vi "_API_BINANCE_GET_USDT_FUTURES_CurrentAllOpenOrders.vi"(0 "BinanceAPI in":refnum<class "BinanceAPI_.lvclass">, 5 "CurrentAllOpenOrders":cluster{"symbol (eg. BTCUSDT)":string}, 11 "error in (no error)":errorcluster) -> (4 "BinanceAPI out":refnum<class "BinanceAPI_.lvclass">, 14 "Body":string, 15 "error out":errorcluster)   [LabVIEW 2022 SP3, in "BinanceAPI_.lvclass"]
doc: "https://binance-docs.github.io/apidocs/futures/en/#current-all-open-orders-user_data"
uses:
  BinanceAPI_.lvclass
  BinanceAPI_.lvclass/BinanceAPI_.ctl
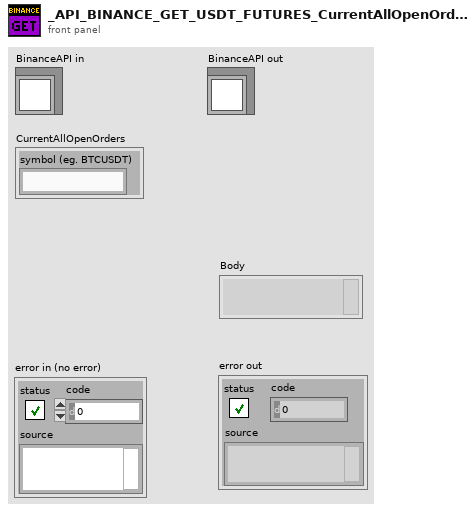
[diagram p1: front panel]
types:
  T1 = enum16{"SPOT", "USDT_FUTURES", "COIN_FUTURES", "VANILLA"}
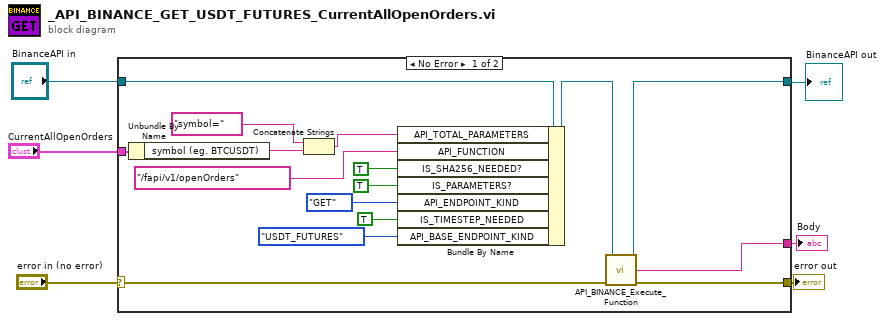
[diagram p0: block diagram]
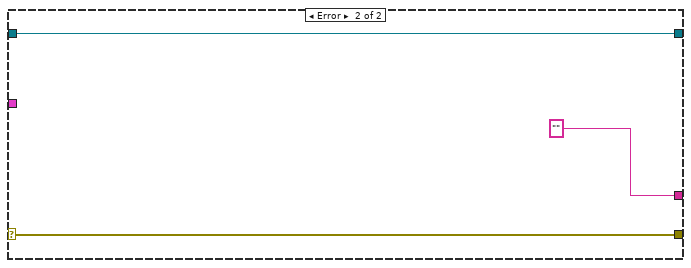
[diagram p2: hidden frame]
diagram:
  n1 = case shown="No Error" "error in (no error)" {
    selector: "error in (no error)" -> [w11 w25]
    tunnel: [w10 w25] -> w4
    tunnel: [w12 w24] -> w1
    tunnel: "BinanceAPI in" -> [w22 w24]
    tunnel: "CurrentAllOpenOrders" -> [w15 _]
    tunnel: [w7 "" ("Header")] -> w3
    frame No Error {
      n2 = Unbundle By Name(w15) -> ("symbol (eg. BTCUSDT)"=w14:string)
      n3 = Concatenate Strings("symbol=", w14) -> (w16:string)
      n4 = Bundle By Name(cluster=w22, "API_TOTAL_PARAMETERS"=w16, "API_FUNCTION"="/fapi/v1/openOrders", "IS_SHA256_NEEDED?"=TRUE, "IS_PARAMETERS?"=TRUE, "API_ENDPOINT_KIND"=enum16{"POST", "DELETE", "GET", "PUT"}."GET", "IS_TIMESTEP_NEEDED"=TRUE, "API_BASE_ENDPOINT_KIND"=T1."USDT_FUTURES") -> (w13:refnum<class "BinanceAPI_.lvclass">)
      n5 = call "API_BINANCE_Execute_Function.vi"("BinanceAPI in"=w13, "error in (no error)"=w11) -> ("BinanceAPI out"=w12:refnum<class "BinanceAPI_.lvclass">, "Body"=w7:string, "error out"=w10:errorcluster)  [unwired: 9 in, 2 out]
    }
    frame Error {
    }
  }
  "error out" <- w4
  "Body" <- w3
  "BinanceAPI out" <- w1
